vi "EMV Slope Flow Detector.vi"(8 "error in (no error)":errorcluster, 11 "Current T6 Temperatures in":dbl[](array[numeric])) -> (0 "error out":errorcluster, 1 "slope":dbl, 3 "Current T6 Temperatures out":dbl[](array[numeric]))   [LabVIEW 2016]
uses:
  <vilib>/Analysis/6fits.llb/Curve Fitting Criteria.ctl
  <vilib>/Analysis/NI_AALPro.lvlib
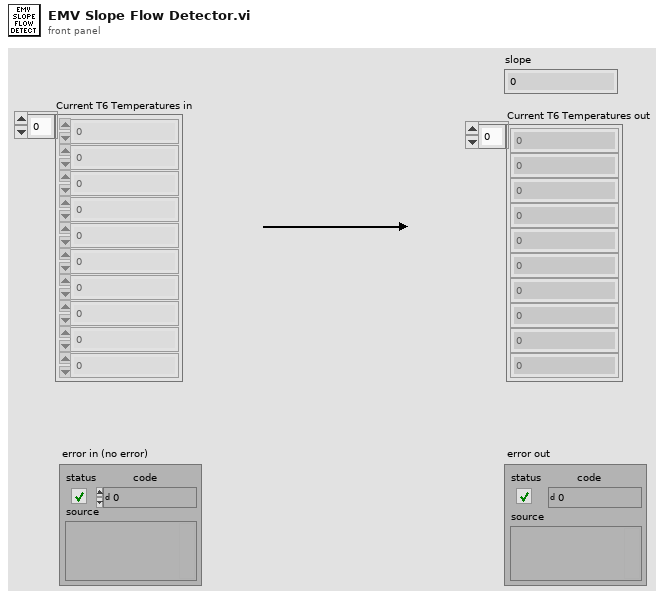
[diagram p1: front panel]
types:
  T1 = typedef "NI_AALPro.lvlib/Curve Fitting Criteria.ctl" = u16
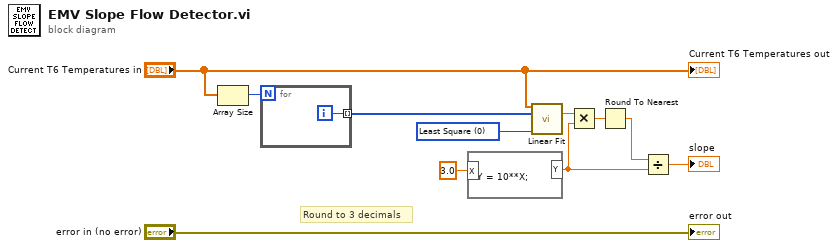
[diagram p0: block diagram]
diagram:
  w11 = T1 0 items=["Least Square", "Least Absolute Residual", "Bisquare"] ("method")
  # "Round to 3 decimals"
  n1 = Array Size(array="Current T6 Temperatures in") -> (size(s)=w9:i32)
  n2 = for {
    N: w9 -> [_]
    tunnel: [w12] -> w10 mode=indexing
    i -> [w12]
  }
  n3 = formula code="Y = 10**X;"("X"=3.0) -> ("Y"=w3:dbl)
  n4 = call <vilib>:"Linear Fit.vi"("Y"="Current T6 Temperatures in", "X"=w10, "method"=w11) -> ("slope"=w2:dbl)  [unwired: 8 in, 4 out]
  n5 = Multiply(x=w2, y=w3) -> (x*y=w5:dbl)
  n6 = Round To Nearest(number=w5) -> (nearest integer value=w4:dbl)
  n7 = Divide(x=w4, y=w3) -> (x/y=→"slope":dbl)
  "error out" <- "error in (no error)"
  "Current T6 Temperatures out" <- "Current T6 Temperatures in"
